vi "Read word (1).vi"() -> ()   [LabVIEW 2021]
panel:
  out "ArrayOut 2":string[](array[string])
  out "Output String Array 2":string[][](array[string])
  in  "stop":bool
  in  "Path":path
  out "Text":string
  in  "Word._Application":refnum<k7>
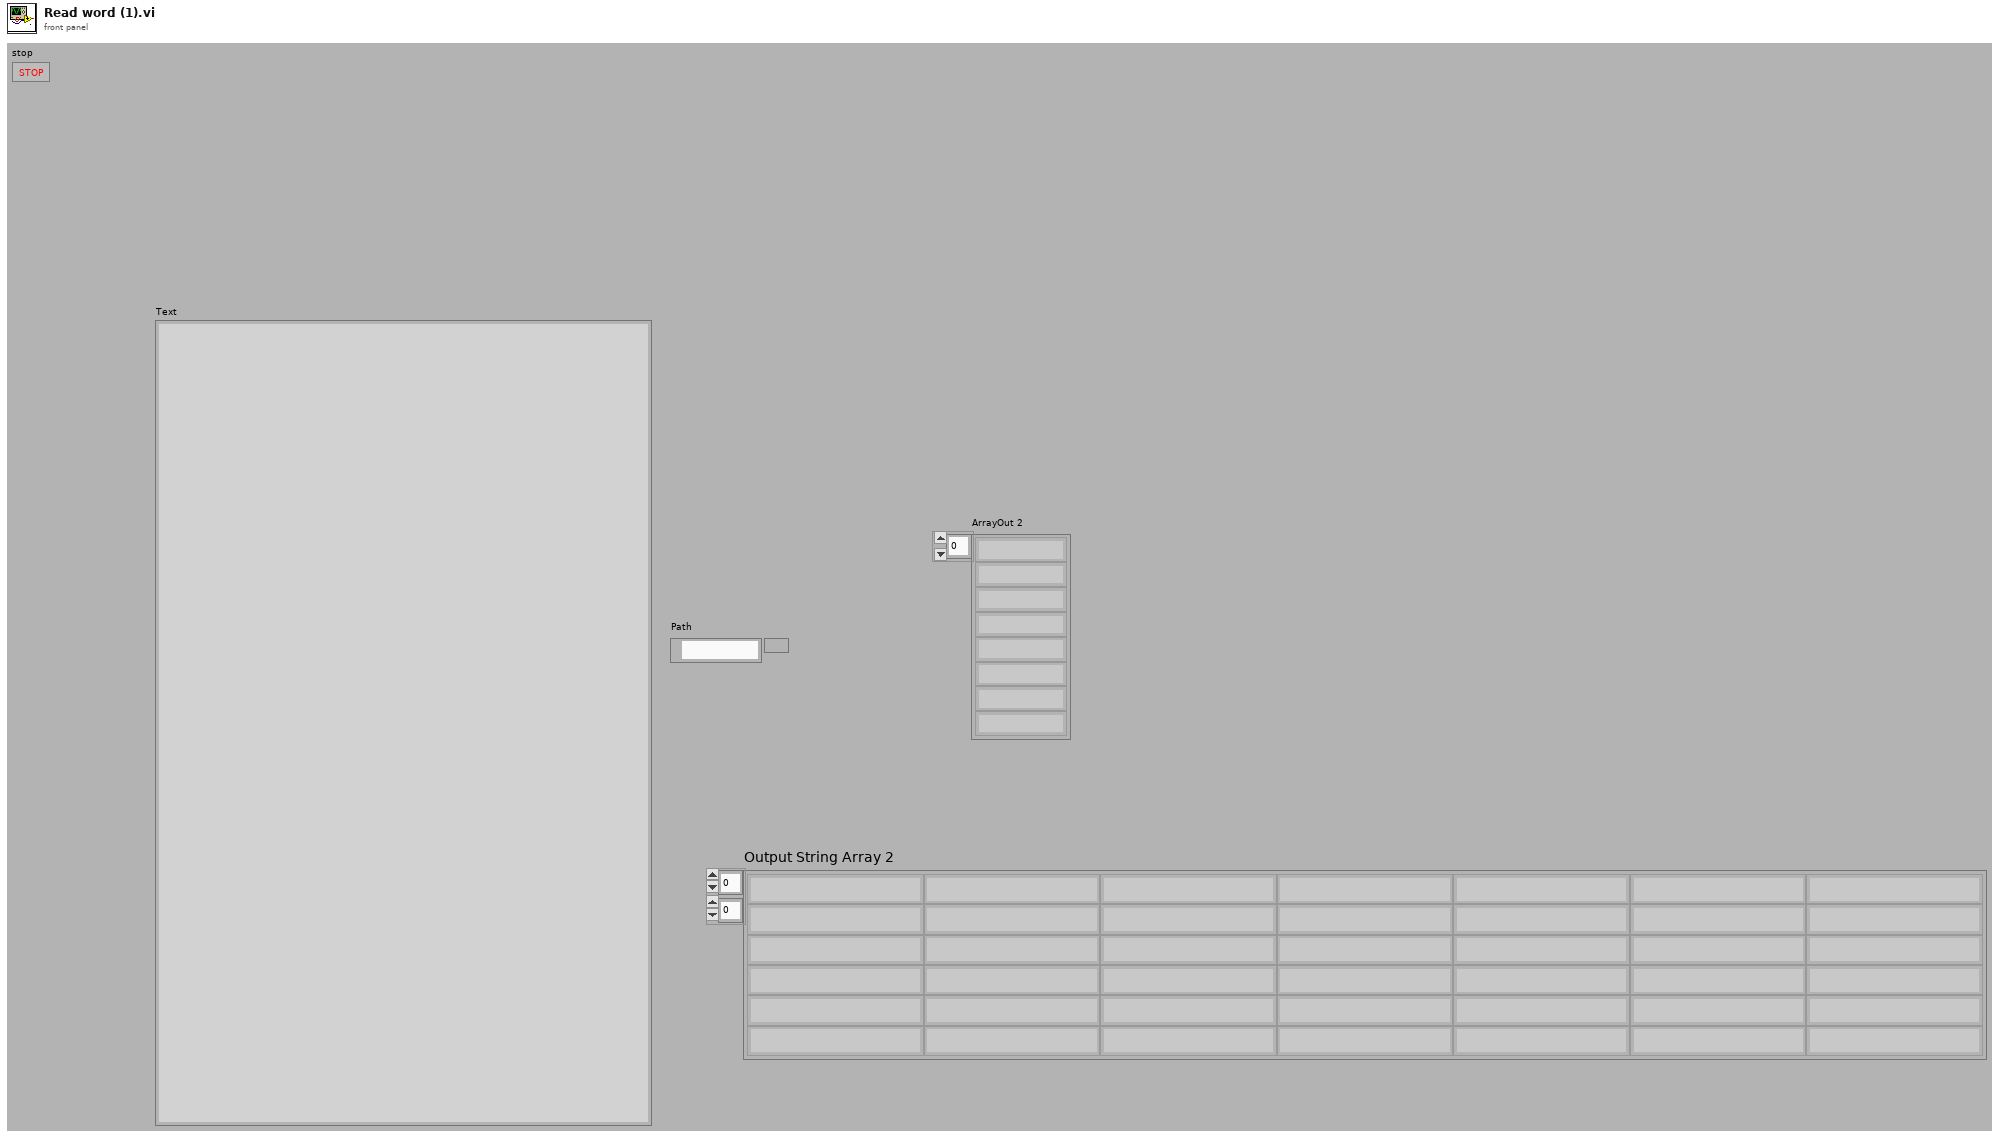
[diagram p1: front panel]
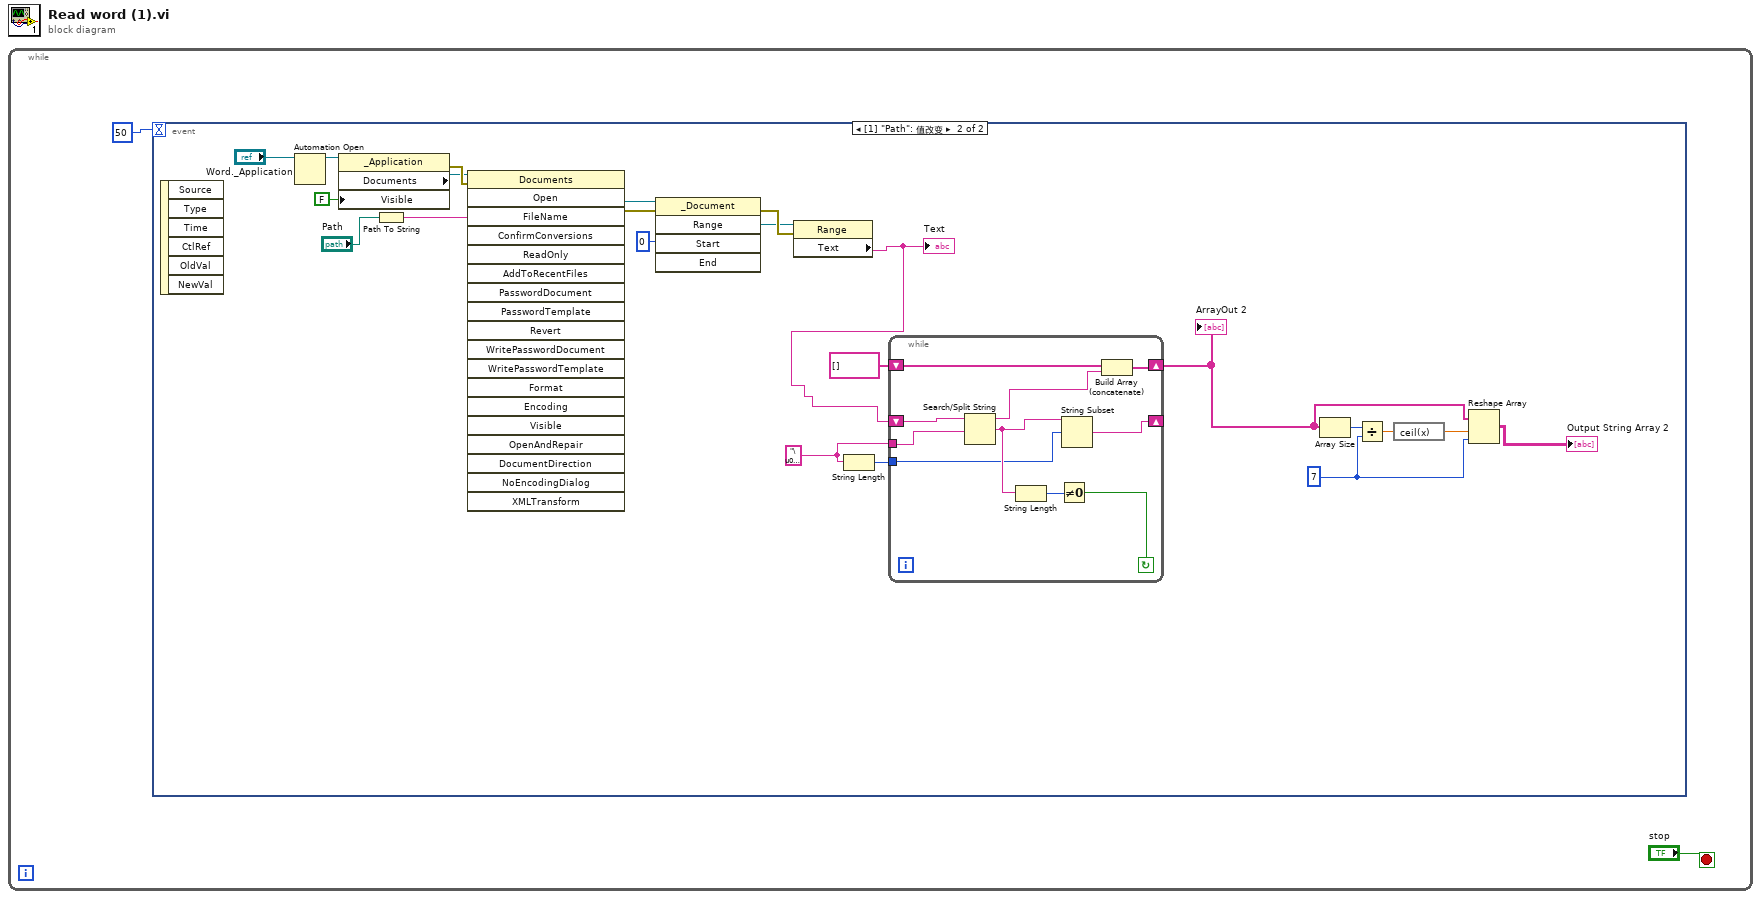
[diagram p0: block diagram]
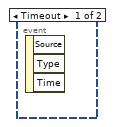
[diagram p2: hidden frame]
diagram:
  n1 = while {
    stop <- "stop" stop-if-true
    n2 = event shown="[1] \"Path\": 值改变" {
      selector: _ -> [_ _]
      dyn-events: _ -> [_ _]
      timeout: 50 -> [_ _]
      event Timeout {
        n3 = event-data() -> ()  [unwired: 1 in, 3 out]
      }
      event "Path": Value Change {
        w12 = "\u0007" ("字符串")
        w11 = 7 ("维数大小")
        n4 = event-data() -> ()  [unwired: 1 in, 6 out]
        n5 = Automation Open(Automation Refnum="Word._Application") -> (Automation Refnum=w15:refnum<k7>)  [unwired: 3 in, 1 out]
        n6 = property class="_Application"(reference=w15, "Visible"=FALSE) -> (error out=w17:errorcluster, "Documents"=w16:refnum<k7>)  [unwired: 1 in, 1 out]
        n7 = Path To String(path="Path") -> (string=w18:string)
        n8 = invoke class="Documents" method="Open"(reference=w16, error in=w17, "FileName"=w18) -> (error out=w21:errorcluster, "Open"=w19:refnum<k7>)  [unwired: 16 in, 17 out]
        n9 = invoke class="_Document" method="Range"(reference=w19, error in=w21, "Start"=0) -> (error out=w22:errorcluster, "Range"=w20:refnum<k7>)  [unwired: 2 in, 3 out]
        n10 = property class="Range"(reference=w20, error in=w22) -> ("Text"=w3:string)  [unwired: 2 out]
        "Text" <- w3
        n11 = String Length(string=w12) -> (length=w5:i32)
        n12 = while {
          tunnel: w5 -> [w25]
          shift-left: string[] [] -> [w31]
          shift-right: [w32] -> w9
          shift-left: w3 -> [w33]
          shift-right: [w30] -> _
          tunnel: w12 -> [w34]
          stop <- w26 continue-if-true
          n13 = Search/Split String(string=w33, search string/char (-)=w34) -> (substring before match=w29:string, match + rest of string=w28:string)  [unwired: 1 in, 1 out]
          n14 = String Length(string=w28) -> (length=w27:i32)
          n15 = Not Equal To 0?(x=w27) -> (x != 0?=w26:bool)
          n16 = String Subset(string=w28, offset (0)=w25) -> (substring=w30:string)  [unwired: 1 in]
          n17 = Build Array (concatenate)(w31, w29) -> (w32:string[])
        }
        "ArrayOut 2" <- w9
        n18 = Array Size(array=w9) -> (size(s)=w8:i32)
        n19 = Divide(x=w8, y=w11) -> (x/y=w7:dbl)
        n20 = expression code="ceil(x)"(w7) -> (w6:dbl)
        n21 = Reshape Array(w9, w6, w11) -> (→"Output String Array 2":string[][])
      }
    }
  }
